vi "main.vi"() -> ()   [LabVIEW 2021]
uses:
  13197e2e-4878-48b7-aae8-aaf27b3d4d67.vi
  0f9acb16-a936-4ed4-a93c-6b467a9371f4.vi
  96cf3d6d-d879-4930-96c0-5a5e60d91763.vi
  Global.vi
  <vilib>/Utility/file.llb/Read Delimited Spreadsheet (DBL).vi
  <vilib>/addons/_NISVFA/_Generation/SoundVib_Generation.lvlib
  <vilib>/measure/NI_MABase.lvlib
panel:
  in  "开始测试":bool
  in  "Stop":bool
  in  "起始频率[Hz]":dbl=1.0 min=1.0 step=100.0
  in  "终止频率[Hz]":dbl=1.0 min=1.0 step=100.0
  in  "信号幅值[V]":dbl min=0.0001 step=0.1
  in  "单次信号时长[s]":dbl
  in  "应用":bool
  in  "Save Button":bool
  in  "Buffer":T1={"# buffers"=4, "Buffer size"=2048, "unit (ms)"=enum."Samples"}
  out "format":cluster{"Rate":i32, "Bits":i32, "Channels":u32}
  out "Waveform Graph":dbl[](graph) caption="Waveform Graph - Dark"
  out "Waveform Graph 3":i32[][](graph)
  out "error out 3":errorcluster
  out "error out":errorcluster
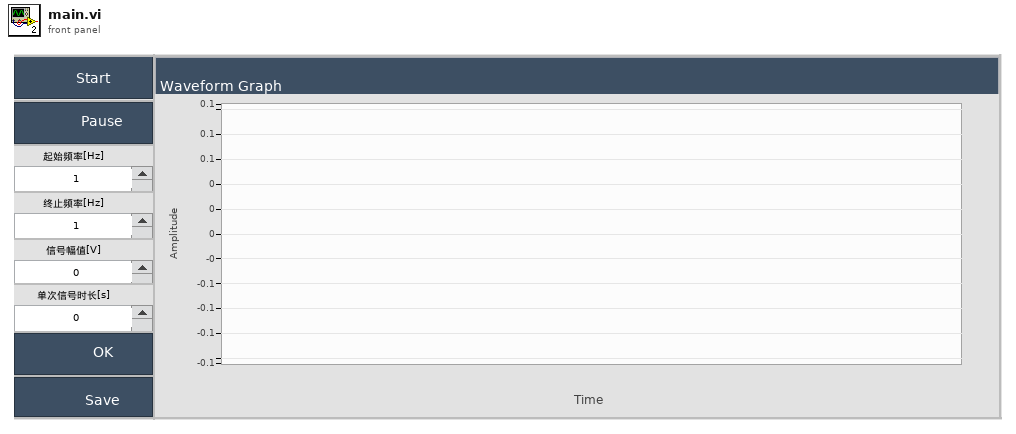
[diagram p1: front panel]
types:
  T1 = cluster{"# buffers":i32, "Buffer size":i32, "unit (ms)":enum16{"time (ms)", "Samples"}}
  T2 = cluster{"slope":dbl, "intercept":dbl, "校准电压值":dbl[]}
  T3 = cluster{"start frequency [Hz]":dbl, "stop frequency [Hz]":dbl}
  T4 = typedef "SoundHandle.ctl" = cluster{"DeviceID":u16, "Samples/buf":u32, "Sampl rate":u32, "Bits/sample":u16, "Channels":u8, "Opened":bool}
  T5 = cluster{"起始频率":dbl, "终止频率":dbl, "信号幅值":dbl, "信号时长":dbl, "重复次数":i32, "扫频模式":bool}
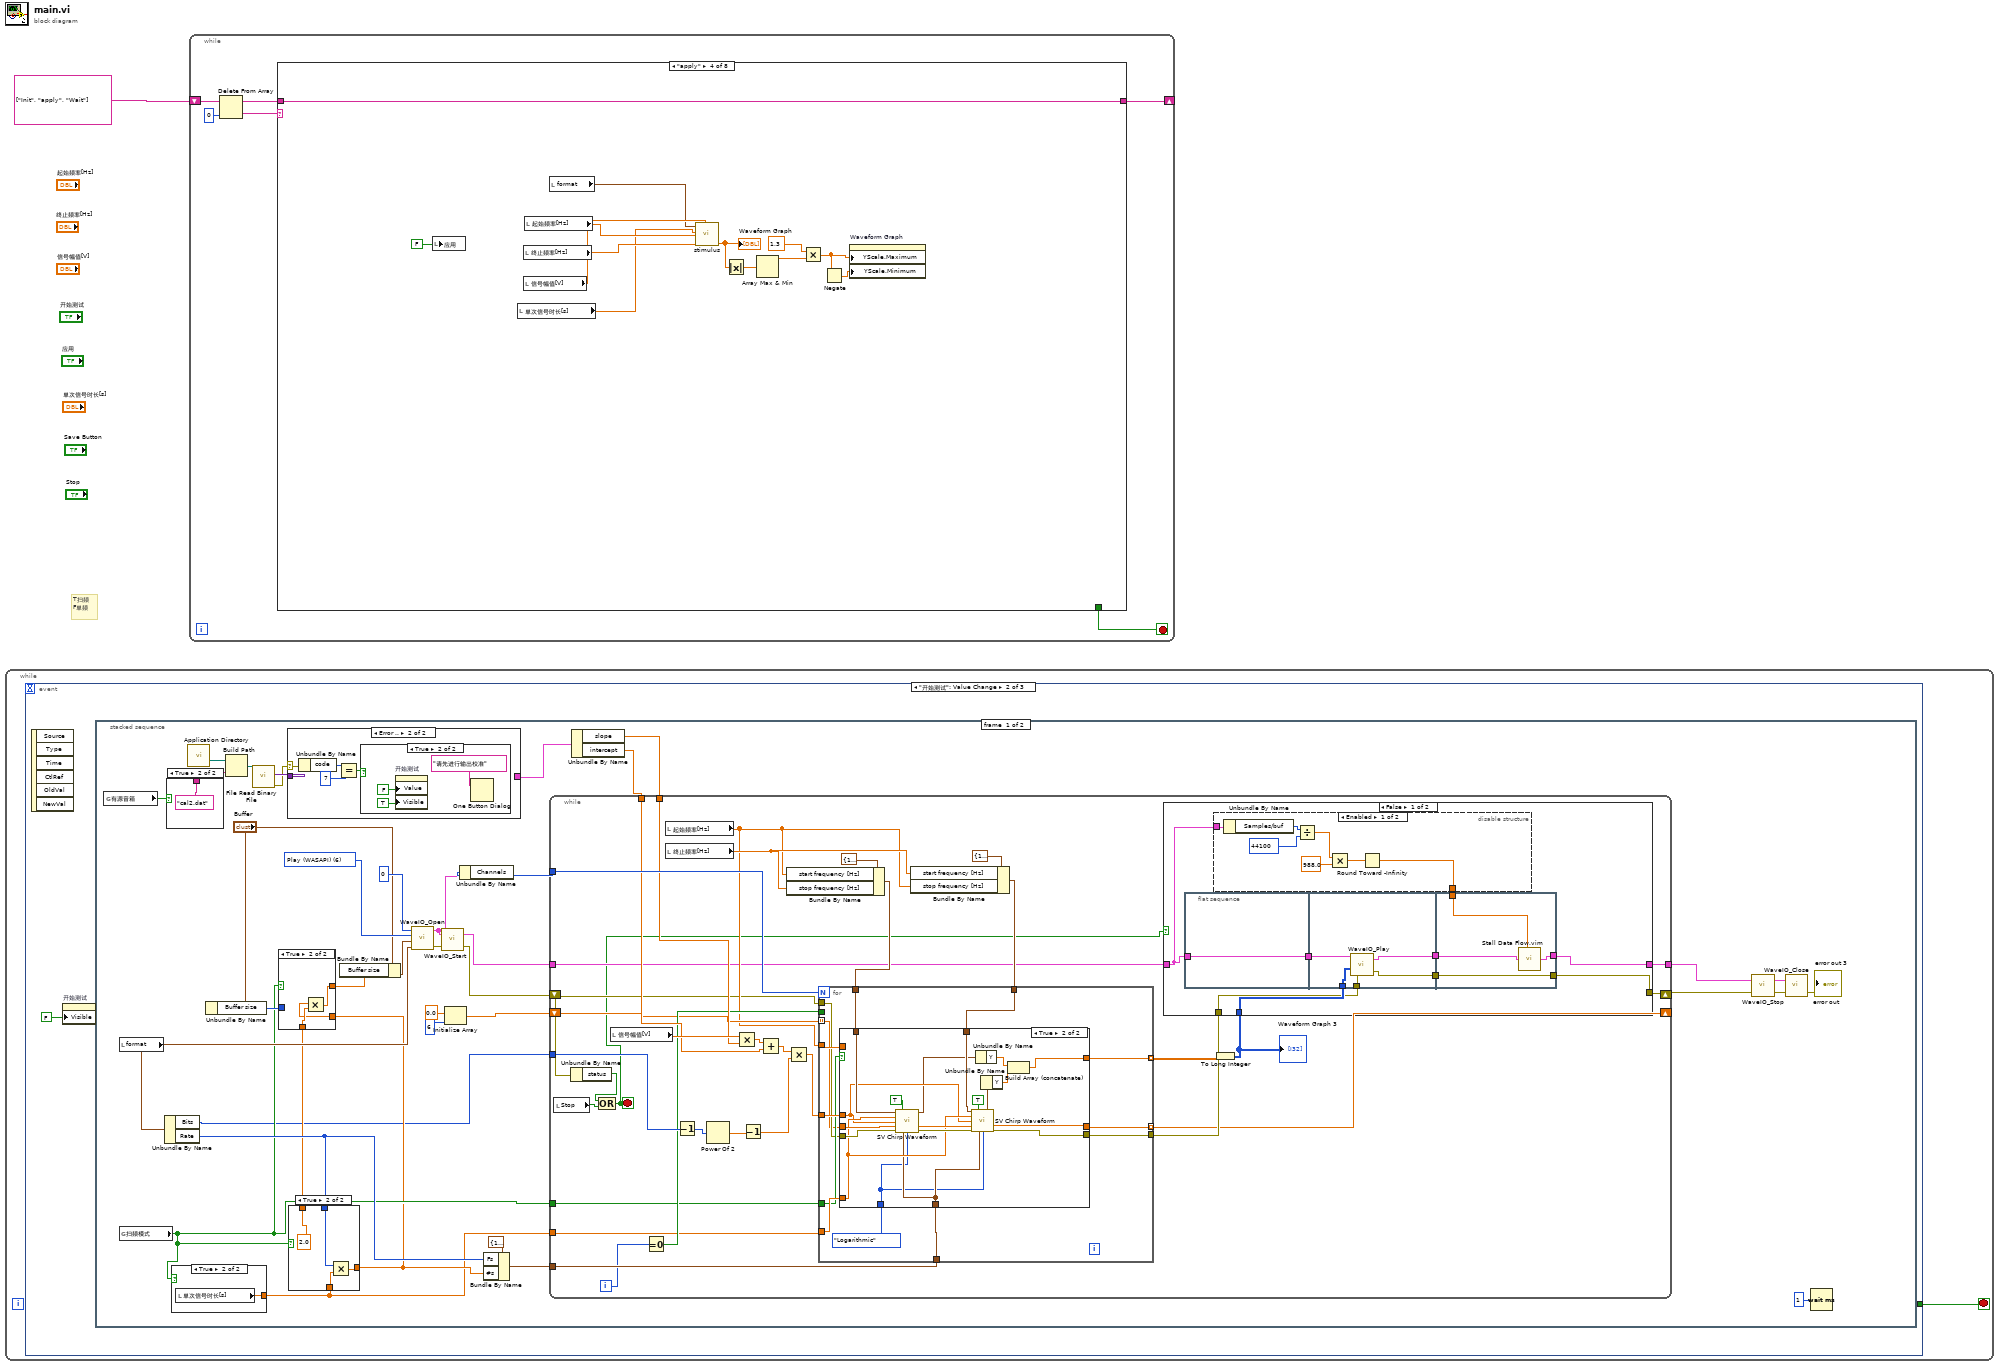
[diagram p0: block diagram]
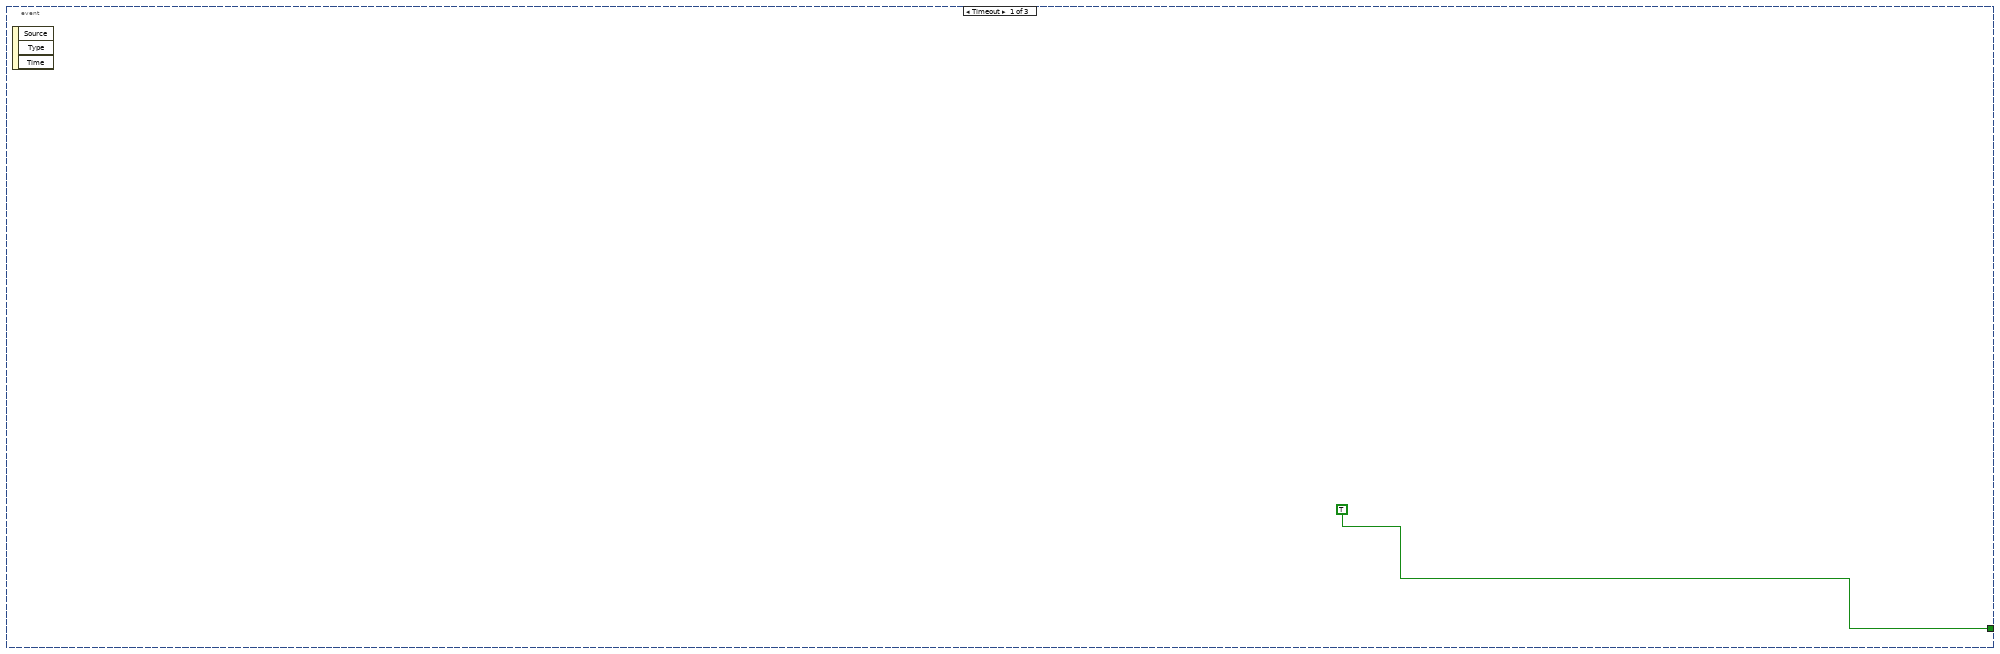
[diagram p2: hidden frame]
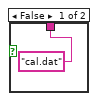
[diagram p3: hidden frame]
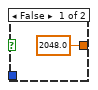
[diagram p4: hidden frame]
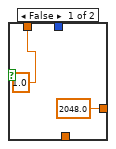
[diagram p5: hidden frame]
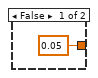
[diagram p6: hidden frame]
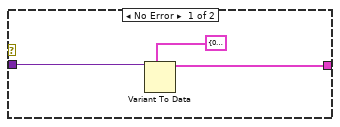
[diagram p7: hidden frame]
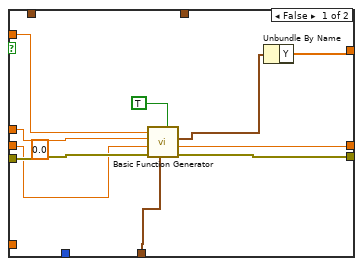
[diagram p11: hidden frame]
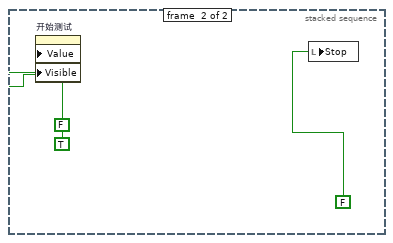
[diagram p12: hidden frame]
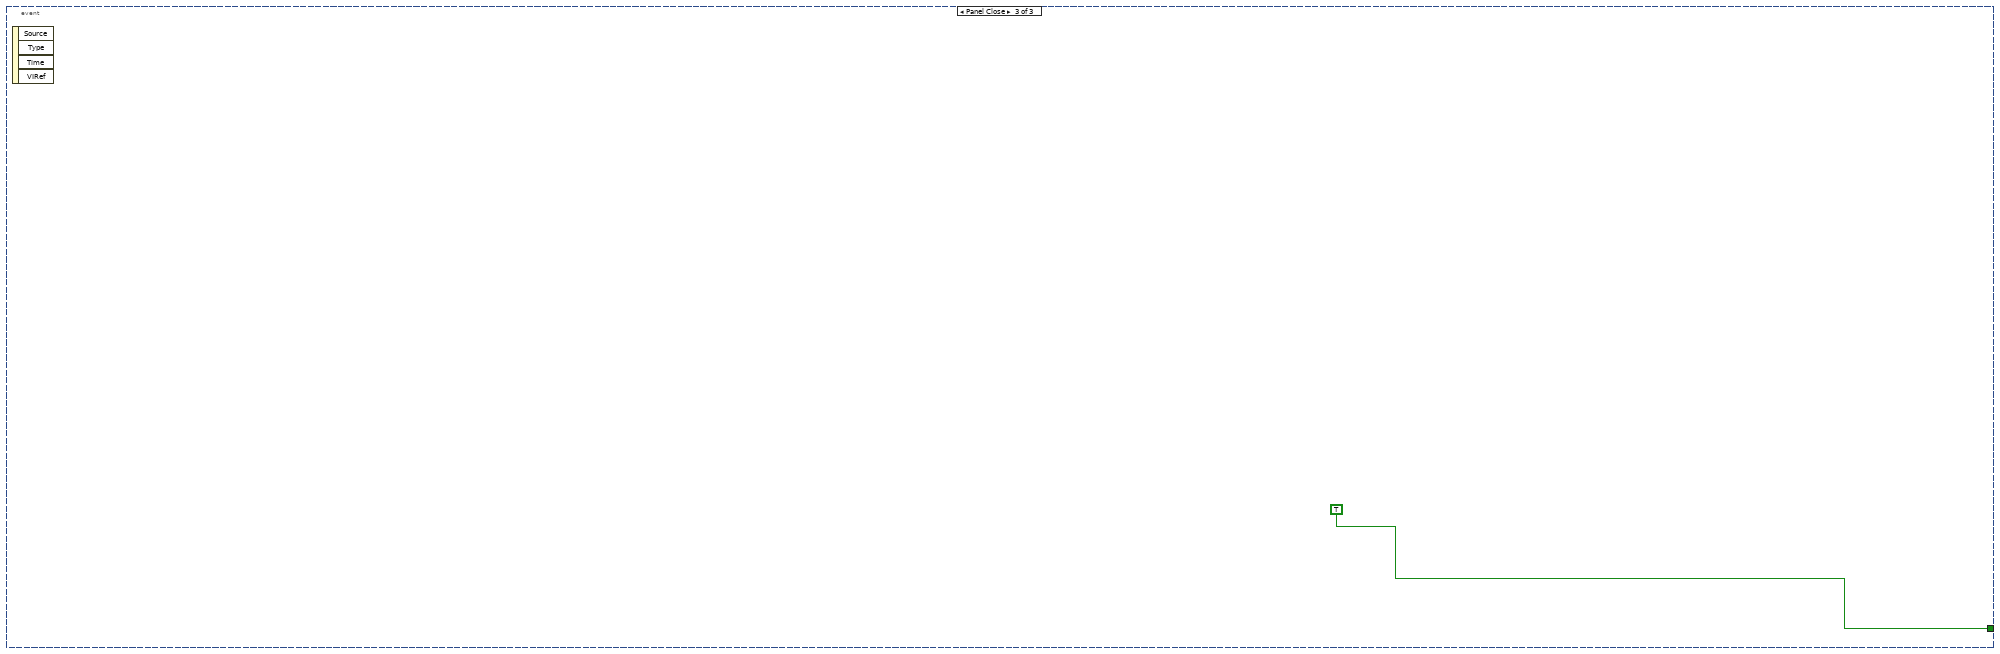
[diagram p13: hidden frame]
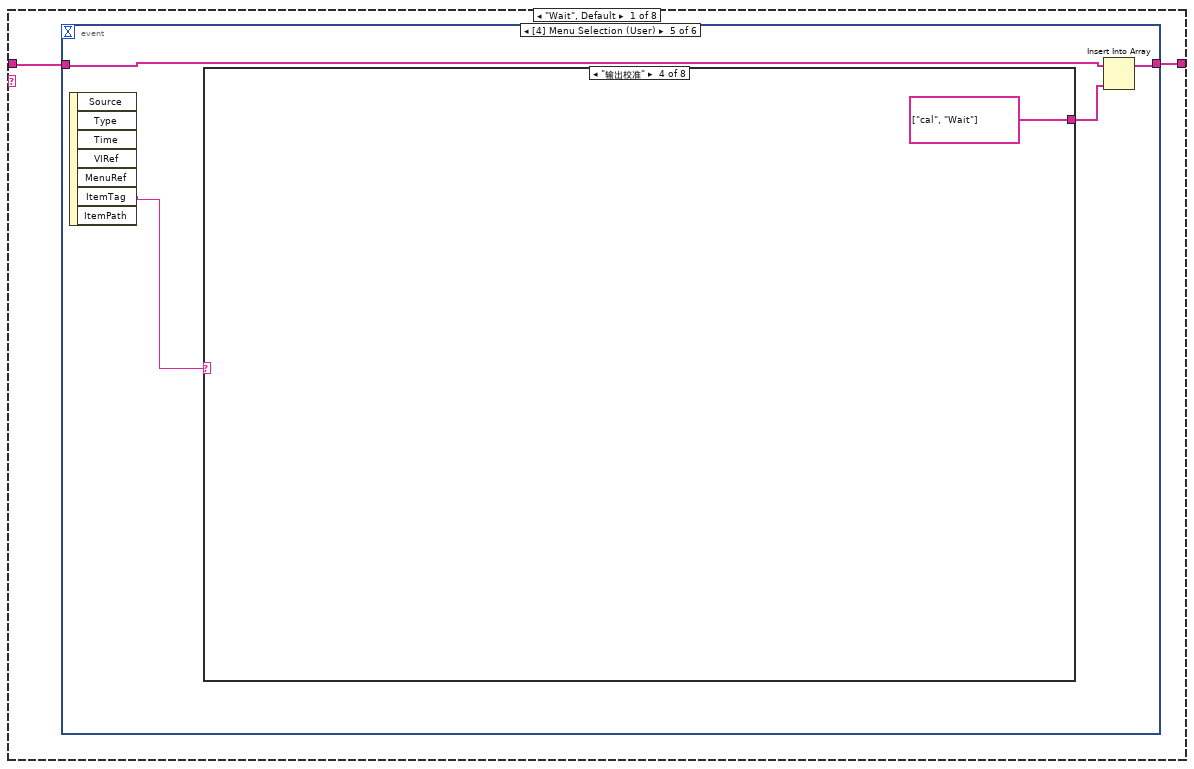
[diagram p14: hidden frame]
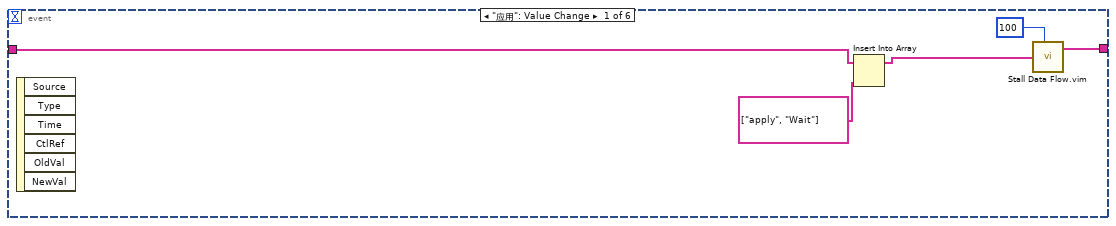
[diagram p15: hidden frame]
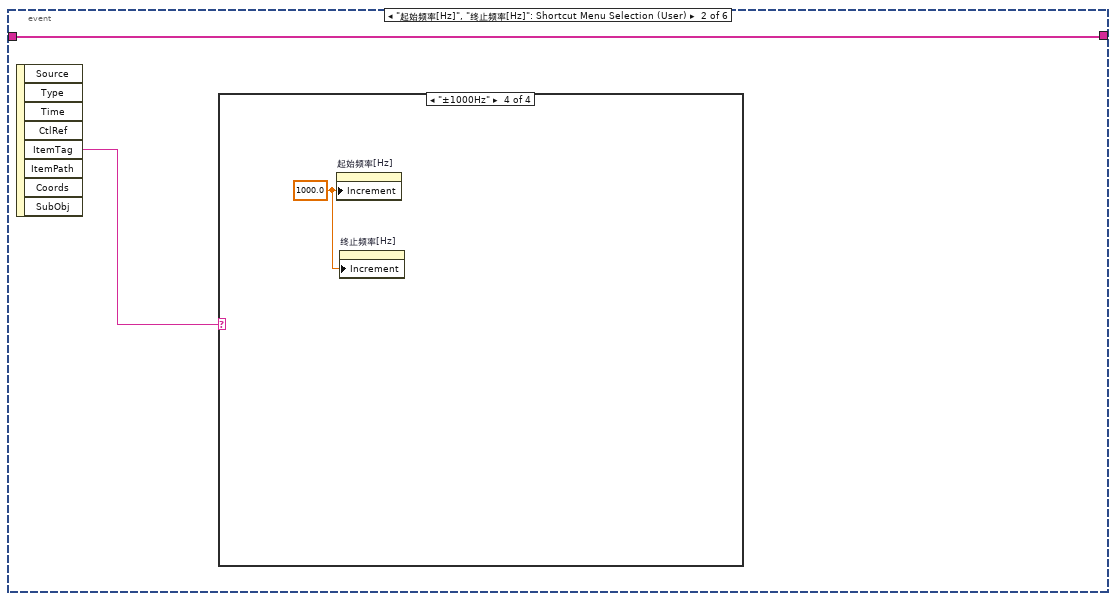
[diagram p16: hidden frame]
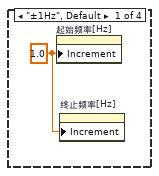
[diagram p17: hidden frame]
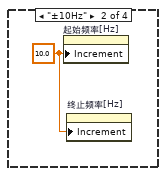
[diagram p18: hidden frame]
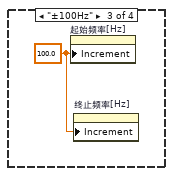
[diagram p19: hidden frame]
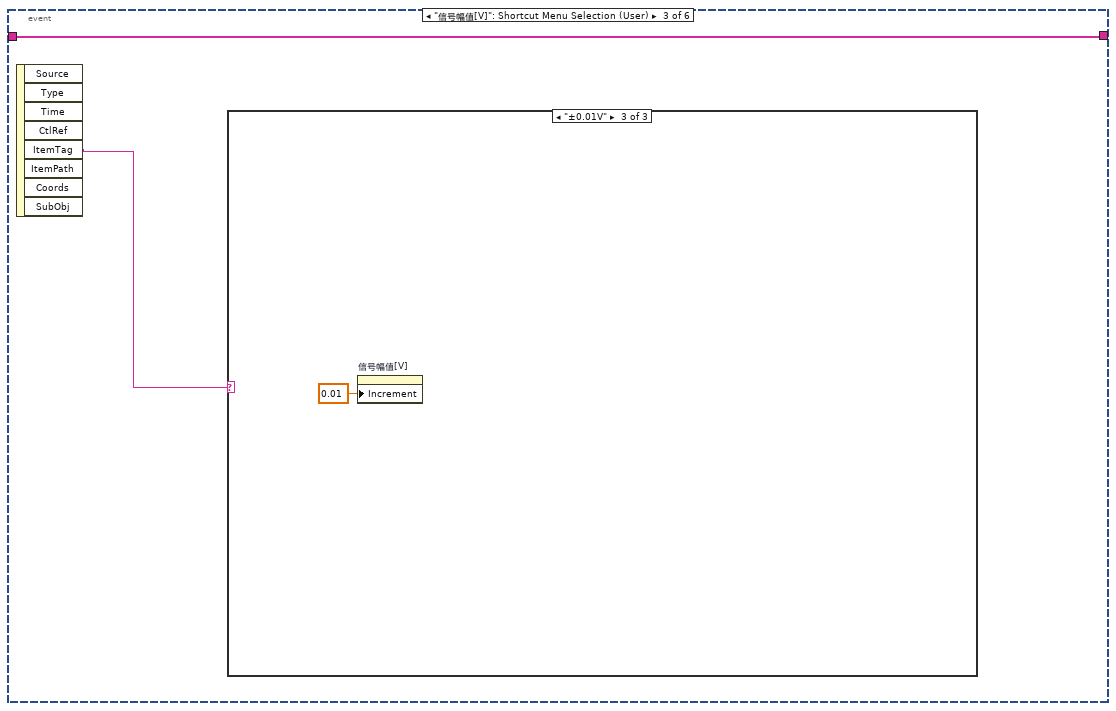
[diagram p20: hidden frame]
diagram:
  # "T扫频\nF单频"
  n1 = while {
    stop <- w2 stop-if-true
    n2 = event shown="[1] \"开始测试\": Value Change" {
      selector: _ -> [_ _ _]
      dyn-events: _ -> [_ _ _]
      timeout: _ -> [_ _ _]
      tunnel: [TRUE ("放弃？") _ TRUE ("放弃？")] -> w2
      event Timeout {
        n3 = event-data() -> ()  [unwired: 1 in, 3 out]
      }
      event "开始测试": Value Change {
        n4 = event-data() -> ()  [unwired: 1 in, 6 out]
        n5 = property on="开始测试" class="Bool (strict)"("Visible"=FALSE) -> ()  [unwired: 2 in, 2 out]
        n6 = stacked-sequence {
          frame #0 {
            w27 = u16 6 items=["Record", "Play", "Loopback", "ASIO input", "ASIO output", "Record (WASAPI)", "Play (WASAPI)", "Record Combi", "Play Combi"] ("device type (Record)")
            n7 = global read "Global.vi" "有源音箱"() -> (w5:bool)
            n8 = local read "format"() -> (w42:cluster{"Rate":i32, "Bits":i32, "Channels":u32})
            n9 = global read "Global.vi" "扫频模式"() -> (w9:bool)
            n10 = Unbundle By Name(w42) -> ("Bits"=w6:i32, "Rate"=w15:i32)
            n11 = case shown="True" w5 {
              tunnel: ["cal.dat" ("名称或相对路径") "cal2.dat" ("名称或相对路径")] -> w26
              frame False {
              }
              frame True {
              }
            }
            n12 = case shown="True" w9 {
              tunnel: [0.05 ("单次信号时长[s]") w57] -> w7
              frame False {
              }
              frame True {
                n13 = local read "单次信号时长[s]"() -> (w57:dbl)
              }
            }
            n14 = call <vilib>:"Application Directory.vi"() -> ("Application Directory"=w25:path)
            n15 = Unbundle By Name("Buffer") -> ("Buffer size"=w10:i32)
            n16 = Build Path(base path=w25, name or relative path=w26) -> (appended path=w24:path)
            n17 = call "File Read Binary File.vi"("file path"=w24) -> ("error Output"=w19:errorcluster, "Variant Output"=w23:variant)  [unwired: 8 in, 1 out]
            n18 = case shown="Error .." w19 {
              selector: w19 -> [_ w64]
              tunnel: w23 -> [w60 _]
              tunnel: [w59 _] -> w22
              frame No Error {
                n19 = Variant To Data(type=T2 {"slope"=0.0, "intercept"=0.0, "校准电压值"=[3.37, 6.73, 10.1, 13.48]}, Variant=w60) -> (data=w59:T2)  [unwired: 1 in, 1 out]
              }
              frame Error {
                n20 = Unbundle By Name(w64) -> ("code"=w63:i32)
                n21 = Equal?(x=w63, y=7) -> (x = y?=w61:bool)
                n22 = case shown="True" w61 {
                  frame False {
                  }
                  frame True {
                    n23 = property on="开始测试" class="Bool (strict)"("Value"=FALSE ("开始测试"), "Visible"=TRUE) -> ()  [unwired: 2 in, 2 out]
                    n24 = One Button Dialog(message="请先进行输出校准") -> ()  [unwired: 1 in, 1 out]
                  }
                }
              }
            }
            n25 = case shown="True" w9 {
              tunnel: [2048.0 w54] -> w8
              tunnel: w7 -> [_ w52]
              tunnel: w15 -> [_ w53]
              tunnel: [1.0 ("x") 2.0 ("x")] -> w11
              frame False {
              }
              frame True {
                n26 = Multiply(x=w53, y=w52) -> (x*y=w54:dbl)
              }
            }
            n27 = case shown="True" w9 {
              tunnel: [2048.0 w47] -> w12
              tunnel: w11 -> [_ w49]
              tunnel: w10 -> [_ _]
              tunnel: w8 -> [_ w48]
              frame False {
              }
              frame True {
                n28 = Multiply(x=w48, y=w49) -> (x*y=w47:dbl)
              }
            }
            n29 = Bundle By Name(cluster="Buffer", "Buffer size"=w12) -> (w14:T1)
            n30 = call "WaveIO_Open.vi"("idev"=u32 0, "device type (Record)"=w27, "Buffer Config"=w14, "Format (44kHz, 16Bit, stereo)"=w42) -> ("Sound Handle Out"=w38:T4, "error out"=w35:errorcluster)  [unwired: 3 in]
            n31 = call "WaveIO_Start.vi"("error in (no error)"=w35, "Handle"=w38) -> ("error out"=w34:errorcluster, "Handle Out"=w33:T4)
            n32 = Initialize Array(0.0 ("element"), 6 ("dimension size")) -> (w16:dbl[])
            n33 = Unbundle By Name(w38) -> ("Channels"=w39:u8)
            n34 = Bundle By Name(cluster=cluster{"Fs":dbl, "#s":dbl} {"Fs"=1000.0, "#s"=1000.0} ("sampling info"), "Fs"=w15, "#s"=w8) -> (w32:cluster{"Fs":dbl, "#s":dbl})
            n35 = Unbundle By Name(w22) -> ("slope"=w21:dbl, "intercept"=w20:dbl)
            n36 = while {
              shift-right: [w95] -> w36
              shift-left: w34 -> [w70]
              tunnel: w33 -> [w73]
              tunnel: [w100] -> w29
              tunnel: w32 -> [w101]
              tunnel: w6 -> [w99]
              tunnel: w39 -> [w94]
              tunnel: w21 -> [w88]
              tunnel: w20 -> [w86]
              tunnel: w9 -> [w82]
              shift-right: [w79] -> _
              shift-left: w16 -> [w80]
              tunnel: w7 -> [w78]
              i -> [w84]
              stop <- w68 stop-if-true
              n37 = local read "Stop"() -> (w92:bool)
              n38 = Unbundle By Name(w70) -> ("status"=w93:bool)
              n39 = Compound Arithmetic op=OR(w93, w92) -> (w68:bool)
              n40 = local read "信号幅值[V]"() -> (w89:dbl)
              n41 = Equal To 0?(x=w84) -> (x = 0?=w83:bool)
              n42 = local read "起始频率[Hz]"() -> (w75:dbl)
              n43 = local read "终止频率[Hz]"() -> (w76:dbl)
              n44 = Decrement(x=w99) -> (x-1=w98:i32)
              n45 = Power Of 2(x=w98) -> (2^x=w72:dbl)
              n46 = Multiply(x=w89, y=w88) -> (x*y=w87:dbl)
              n47 = Decrement(x=w72) -> (x-1=w71:dbl)
              n48 = Add(x=w87, y=w86) -> (x+y=w85:dbl)
              n49 = Bundle By Name(cluster=T3 {"start frequency [Hz]"=10.0, "stop frequency [Hz]"=10000.0} ("frequency range"), "start frequency [Hz]"=w75, "stop frequency [Hz]"=w76) -> (w90:T3)
              n50 = Multiply(x=w85, y=w71) -> (x*y=w97:dbl)
              n51 = Bundle By Name(cluster=T3 {"start frequency [Hz]"=10.0, "stop frequency [Hz]"=10000.0} ("frequency range"), "start frequency [Hz]"=w76, "stop frequency [Hz]"=w75) -> (w74:T3)
              n52 = for {
                N: w94 -> [_]
                tunnel: w101 -> [w142]
                tunnel: w97 -> [w141]
                tunnel: [w130] -> w69 mode=indexing
                tunnel: w90 -> [w140]
                tunnel: w78 -> [w139]
                tunnel: w83 -> [_]
                tunnel: w82 -> [w137]
                tunnel: w75 -> [w136]
                tunnel: w70 -> [w135]
                tunnel: [w134] -> w81
                tunnel: w80 -> [w133] mode=indexing
                tunnel: [w132] -> w79 mode=indexing
                tunnel: w74 -> [w131]
                n53 = case shown="True" w137 {
                  tunnel: w142 -> [w148 w155]
                  tunnel: w141 -> [w151 w163]
                  tunnel: w140 -> [_ w170]
                  tunnel: w139 -> [_ w164]
                  tunnel: enum16{"Linear", "Logarithmic"}."Logarithmic" ("frequency spacing") -> [_ w154]
                  tunnel: w136 -> [w152 _]
                  tunnel: w135 -> [w150 w169]
                  tunnel: [w149 w168] -> w134
                  tunnel: w133 -> [w146 w166]
                  tunnel: [w147 w160] -> w132
                  tunnel: w131 -> [_ w162]
                  tunnel: [w143 w153] -> w130
                  frame False {
                    (unwired) 0.0 ("phase")
                    n54 = call <vilib>:"Basic Function Generator.vi"("reset signal"=TRUE, "sampling info"=w148, "error in (no error)"=w150, "phase"=w146, "amplitude"=w151, "frequency"=w152) -> ("error out"=w149:errorcluster, "phase out"=w147:dbl, "signal out"=w145:waveform(dbl))  [unwired: 3 in]
                    n55 = Unbundle By Name(w145) -> ("Y"=w143:dbl[])
                  }
                  frame True {
                    n56 = call <vilib>:"SV Chirp Waveform.vi"("frequency range"=w170, "reset signal (F)"=TRUE, "chirp duration [s]"=w164, "amplitude"=w163, "phase in [deg]"=w166, "error in (no error)"=w169, "sampling info"=w155, "frequency spacing"=w154) -> ("chirp signal"=w159:waveform(dbl), "phase out [deg]"=w165:dbl, "error out"=w168:errorcluster)  [unwired: 5 in]
                    n57 = call <vilib>:"SV Chirp Waveform.vi"("frequency range"=w162, "reset signal (F)"=TRUE, "chirp duration [s]"=w164, "amplitude"=w163, "phase in [deg]"=w165, "sampling info"=w155, "frequency spacing"=w154) -> ("chirp signal"=w158:waveform(dbl), "phase out [deg]"=w160:dbl)  [unwired: 6 in, 1 out]
                    n58 = Unbundle By Name(w159) -> ("Y"=w157:dbl[])
                    n59 = Unbundle By Name(w158) -> ("Y"=w156:dbl[])
                    n60 = Build Array (concatenate)(w157, w156) -> (w153:dbl[])
                  }
                }
              }
              n61 = To Long Integer(number=w69) -> (32bit integer=w96:i32[][])
              "Waveform Graph 3" <- w96
              n62 = case shown="False" w68 {
                tunnel: [w103 w129] -> w100
                tunnel: w96 -> [w110 _]
                tunnel: [w109 w128] -> w95
                tunnel: w81 -> [w108 w128]
                tunnel: w73 -> [w105 w129]
                frame False {
                  n63 = flat-sequence {
                    tunnel: w105 -> [w111]
                    tunnel: [w111] -> w104
                    tunnel: w110 -> [w116]
                    tunnel: w108 -> [w114]
                    tunnel: [w115] -> w107
                    tunnel: [w113] -> w106
                    tunnel: w104 -> [w112]
                    tunnel: w107 -> [w120]
                    tunnel: w106 -> [w118]
                    tunnel: w102 -> [w117]
                    tunnel: [w120] -> w109
                    tunnel: [w119] -> w103
                    frame #0 {
                    }
                    frame #1 {
                      n64 = call "WaveIO_Play.vi"("error in (no error)"=w114, "data"=w116, "Handle"=w112) -> ("error out"=w115:errorcluster, "Handle Out"=w113:T4)  [unwired: 1 in]
                    }
                    frame #2 {
                      n65 = call "Stall Data Flow.vim"("value in"=w118, "milliseconds to wait"=w117) -> ("value out"=w119:T4)  [unwired: 1 out]
                    }
                  }
                  n66 = disable-structure shown="Enabled" {
                    disable-tunnel: w105 -> [w125 _]
                    disable-tunnel: [w121 _] -> w102
                    frame Enabled {
                      n67 = Unbundle By Name(w125) -> ("Samples/buf"=w127:u32)
                      n68 = Divide(x=w127, y=u32 44100) -> (x/y=w124:dbl)
                      n69 = Multiply(x=w124, y=988.0) -> (x*y=w122:dbl)
                      n70 = Round Toward -Infinity(1:w122) -> (0:w121:dbl)
                    }
                    frame Disabled {
                    }
                  }
                }
                frame True {
                }
              }
            }
            n71 = call "WaveIO_Stop.vi"("error in (no error)"=w36, "Handle"=w29) -> ("error out"=w30:errorcluster, "Handle Out"=w28:T4)
            n72 = call "WaveIO_Close.vi"("error in (no error)"=w30, "Handle"=w28) -> ("error out"=→"error out 3":errorcluster)  [unwired: 1 out]
            n73 = Wait (ms)(milliseconds to wait=u32 1) -> ()  [unwired: 1 out]
            n74 = Wait (ms)(milliseconds to wait=u32 1) -> ()  [unwired: 1 out]
          }
          frame #1 {
            n75 = property on="开始测试" class="Bool (strict)"("Value"=FALSE ("开始测试"), "Visible"=TRUE) -> ()  [unwired: 2 in, 2 out]
            n76 = local write "Stop"(FALSE ("Stop")) -> ()
          }
        }
      }
      event Panel Close {
        n77 = event-data() -> ()  [unwired: 1 in, 4 out]
      }
    }
  }
  n78 = while {
    shift-right: [w176] -> _
    shift-left: string[] ["Init", "apply", "Wait"] -> [w180]
    stop <- w175 stop-if-true
    n79 = Delete From Array(array=w180, index=0 ("索引")) -> (deleted portion=w178:string, array with subset deleted=w177:string[])  [unwired: 1 in]
    n80 = case shown="\"apply\"" w178 {
      tunnel: w177 -> [w181 w224 w232 w251 w257 w294 w359 w388]
      tunnel: [w182 w224 w232 w251 w257 w295 w359 w388] -> w176
      tunnel: [_ _ _ _ _ _ TRUE _] -> w175
      frame "Wait", Default {
        n81 = event shown="[4] Menu Selection (User)" {
          selector: _ -> [_ _ _ _ _ _]
          dyn-events: _ -> [_ _ _ _ _ _]
          timeout: _ -> [_ _ _ _ _ _]
          tunnel: [w187 w189 w194 w203 w204 w221] -> w182
          tunnel: w181 -> [w185 w189 w194 w201 w206 w223]
          event "应用": Value Change {
            n82 = event-data() -> ()  [unwired: 1 in, 6 out]
            n83 = Insert Into Array(array=w185, new element=string[] ["apply", "Wait"]) -> (w183:string[])  [unwired: 1 in]
            n84 = call "Stall Data Flow.vim"("value in"=w183, "milliseconds to wait"=u32 100) -> ("value out"=w187:string[])  [unwired: 1 out]
          }
          event "起始频率[Hz]", "终止频率[Hz]": Shortcut Menu Selection (User) {
            n85 = event-data() -> ("ItemTag"=w188:string)  [unwired: 1 in, 7 out]
            n86 = case shown="\"±1000Hz\"" w188 {
              frame "±1Hz", Default {
                w190 = 1.0 ("Data Entry Limits:Increment")
                n87 = property on="起始频率[Hz]" class="DigNum (strict)"("Increment"=w190) -> ()  [unwired: 2 in, 2 out]
                n88 = property on="终止频率[Hz]" class="DigNum (strict)"("Increment"=w190) -> ()  [unwired: 2 in, 2 out]
              }
              frame "±10Hz" {
                w191 = 10.0 ("Data Entry Limits:Increment")
                n89 = property on="起始频率[Hz]" class="DigNum (strict)"("Increment"=w191) -> ()  [unwired: 2 in, 2 out]
                n90 = property on="终止频率[Hz]" class="DigNum (strict)"("Increment"=w191) -> ()  [unwired: 2 in, 2 out]
              }
              frame "±100Hz" {
                w192 = 100.0 ("Data Entry Limits:Increment")
                n91 = property on="起始频率[Hz]" class="DigNum (strict)"("Increment"=w192) -> ()  [unwired: 2 in, 2 out]
                n92 = property on="终止频率[Hz]" class="DigNum (strict)"("Increment"=w192) -> ()  [unwired: 2 in, 2 out]
              }
              frame "±1000Hz" {
                w193 = 1000.0 ("Data Entry Limits:Increment")
                n93 = property on="起始频率[Hz]" class="DigNum (strict)"("Increment"=w193) -> ()  [unwired: 2 in, 2 out]
                n94 = property on="终止频率[Hz]" class="DigNum (strict)"("Increment"=w193) -> ()  [unwired: 2 in, 2 out]
              }
            }
          }
          event "信号幅值[V]": Shortcut Menu Selection (User) {
            n95 = event-data() -> ("ItemTag"=w195:string)  [unwired: 1 in, 7 out]
            n96 = case shown="\"±0.01V\"" w195 {
              frame "±1V", Default {
                n97 = property on="信号幅值[V]" class="DigNum (strict)"("Increment"=1.0 ("Data Entry Limits:Increment")) -> ()  [unwired: 2 in, 2 out]
              }
              frame "±0.1V" {
                n98 = property on="信号幅值[V]" class="DigNum (strict)"("Increment"=0.1 ("Data Entry Limits:Increment")) -> ()  [unwired: 2 in, 2 out]
              }
              frame "±0.01V" {
                n99 = property on="信号幅值[V]" class="DigNum (strict)"("Increment"=0.01 ("Data Entry Limits:Increment")) -> ()  [unwired: 2 in, 2 out]
              }
            }
          }
          event "Save Button": Value Change {
            n100 = event-data() -> ()  [unwired: 1 in, 6 out]
            n101 = Insert Into Array(array=w201, new element=string[] ["save", "Wait"]) -> (w199:string[])  [unwired: 1 in]
            n102 = call "Stall Data Flow.vim"("value in"=w199, "milliseconds to wait"=u32 100) -> ("value out"=w203:string[])  [unwired: 1 out]
          }
          event Menu Selection (User) {
            n103 = event-data() -> ("ItemTag"=w207:string)  [unwired: 1 in, 6 out]
            n104 = case shown="\"输出校准\"" w207 {
              tunnel: [_ string[] ["signal out", "Wait"] string[] ["signal in", "Wait"] string[] ["cal", "Wait"] _ _ _ _] -> w205
              frame Default {
              }
              frame "扫频信号导出" {
              }
              frame "扫频信号导入" {
              }
              frame "输出校准" {
              }
              frame "单频" {
                n105 = property on="单次信号时长[s]" class="DigNum (strict)"("Visible"=FALSE) -> ()  [unwired: 2 in, 2 out]
                n106 = property on="终止频率[Hz]" class="DigNum (strict)"("Visible"=FALSE) -> ()  [unwired: 2 in, 2 out]
                n107 = global write "Global.vi" "扫频模式"(FALSE ("扫频模式")) -> ()
                n108 = property on="起始频率[Hz]" class="DigNum (strict)"("Caption.Text"="单频频率[Hz]") -> ()  [unwired: 2 in, 2 out]
              }
              frame "有源音箱" {
                n109 = global write "Global.vi" "有源音箱"(TRUE ("有源音箱")) -> ()
              }
              frame "其它" {
                n110 = global write "Global.vi" "有源音箱"(FALSE ("有源音箱")) -> ()
              }
              frame "扫频" {
                n111 = property on="单次信号时长[s]" class="DigNum (strict)"("Visible"=TRUE) -> ()  [unwired: 2 in, 2 out]
                n112 = property on="终止频率[Hz]" class="DigNum (strict)"("Visible"=TRUE) -> ()  [unwired: 2 in, 2 out]
                n113 = global write "Global.vi" "扫频模式"(TRUE ("扫频模式")) -> ()
                n114 = property on="起始频率[Hz]" class="DigNum (strict)"("Caption.Text"="起始频率[Hz]") -> ()  [unwired: 2 in, 2 out]
              }
            }
            n115 = Insert Into Array(array=w206, new element=w205) -> (w204:string[])  [unwired: 1 in]
          }
          event Panel Close? {
            n116 = event-data() -> ()  [unwired: 1 in, 4 out]
            n117 = Insert Into Array(array=w223, new element="Exit" ("new element/subarray")) -> (w221:string[])  [unwired: 1 in]
            n118 = event-data() -> ()  [unwired: 2 in, 1 out]
          }
        }
      }
      frame "cal" {
        n119 = local read "单次信号时长[s]"() -> (w230:dbl)
        n120 = local read "起始频率[Hz]"() -> (w228:dbl)
        n121 = local read "终止频率[Hz]"() -> (w229:dbl)
        n122 = local read "信号幅值[V]"() -> (w227:dbl)
        n123 = local read "Buffer"() -> (w226:T1)
        n124 = local read "format"() -> (w225:cluster{"Rate":i32, "Bits":i32, "Channels":u32})
        n125 = call "calibration.vi"("信号时长[s]"=w230, "Buffer"=w226, "终止频率[Hz]"=w229, "起始频率[Hz]"=w228, "信号幅值[V]"=w227, "format"=w225) -> ()  [unwired: 10 in]
      }
      frame "save" {
        n126 = local read "单次信号时长[s]"() -> (w238:dbl)
        n127 = global read "Global.vi" "扫频模式"() -> (w231:bool)
        n128 = local read "终止频率[Hz]"() -> (w240:dbl)
        n129 = local read "信号幅值[V]"() -> (w239:dbl)
        n130 = local read "起始频率[Hz]"() -> (w241:dbl)
        n131 = local write "Save Button"(FALSE ("应用")) -> ()
        n132 = Bundle By Name(cluster=T5 {"起始频率"=0.0, "终止频率"=0.0, "信号幅值"=0.0, "信号时长"=0.0, "重复次数"=3, "扫频模式"=TRUE}, "起始频率"=w241, "终止频率"=w240, "信号幅值"=w239, "信号时长"=w238, "扫频模式"=w231) -> (w237:T5)
        n133 = call <vilib>:"Application Directory.vi"() -> ("Application Directory"=w243:path)
        n134 = Build Path(base path=w243, name or relative path="main.dat" ("名称或相对路径")) -> (appended path=w242:path)
        n135 = call "File Write to Variant.vi"("替换提示"=FALSE, "Input Data"=w237, "Path to Write"=w242) -> ()  [unwired: 4 in, 5 out]
      }
      frame "apply" {
        n136 = local write "应用"(FALSE ("应用")) -> ()
        n137 = local read "单次信号时长[s]"() -> (w252:dbl)
        n138 = local read "终止频率[Hz]"() -> (w255:dbl)
        n139 = local read "信号幅值[V]"() -> (w254:dbl)
        n140 = local read "起始频率[Hz]"() -> (w256:dbl)
        n141 = local read "format"() -> (w253:cluster{"Rate":i32, "Bits":i32, "Channels":u32})
        n142 = call "stimulus.vi"("幅值(V)"=w254, "stop frequency [Hz]"=w255, "start frequency [Hz]"=w256, "信号时长"=w252, "Format"=w253) -> ("sti"=w250:dbl[])  [unwired: 4 in, 2 out]
        "Waveform Graph" <- w250
        n143 = Absolute Value(x=w250) -> (abs(x)=w249:dbl[])
        n144 = Array Max & Min(array=w249) -> (max value=w248:dbl)  [unwired: 3 out]
        n145 = Multiply(x=1.3, y=w248) -> (x*y=w245:dbl)
        n146 = Negate(x=w245) -> (-x=w246:dbl)
        n147 = property on="Waveform Graph" class="WFGraph (strict)"("YScale.Maximum"=w245, "YScale.Minimum"=w246) -> ()  [unwired: 2 in, 2 out]
      }
      frame "signal out" {
        n148 = stacked-sequence {
          frame #0 {
            n149 = global read "Global.vi" "扫频模式"() -> (w258:bool)
            n150 = case shown="True" w258 {
              frame True {
                w259 = "Hz" ("string")
                w262 = i16 2 ("precision (6)")
                w261 = "-" ("string")
                w263 = i16 0 ("precision (6)")
                n151 = local read "信号幅值[V]"() -> (w270:dbl)
                n152 = local read "单次信号时长[s]"() -> (w267:dbl)
                n153 = local read "起始频率[Hz]"() -> (w274:dbl)
                n154 = local read "终止频率[Hz]"() -> (w273:dbl)
                n155 = local read "format"() -> (w277:cluster{"Rate":i32, "Bits":i32, "Channels":u32})
                n156 = call "stimulus.vi"("幅值(V)"=w270, "stop frequency [Hz]"=w273, "start frequency [Hz]"=w274, "信号时长"=w267, "Format"=w277) -> ("sti"=w276:dbl[])  [unwired: 4 in, 2 out]
                n157 = Number To Fractional String(number=w274, precision (6)=w263) -> (F-format string=w272:string)  [unwired: 2 in]
                n158 = Number To Fractional String(number=w273, precision (6)=w263) -> (F-format string=w271:string)  [unwired: 2 in]
                n159 = Number To Fractional String(number=w270, precision (6)=w262) -> (F-format string=w269:string)  [unwired: 2 in]
                n160 = Number To Fractional String(number=w267, precision (6)=w262) -> (F-format string=w266:string)  [unwired: 2 in]
                n161 = Concatenate Strings(w272, w259, w261, w271, w259, w261, w269, "V" ("string"), w261, w266, "s" ("string"), ".txt" ("string")) -> (w264:string)
                n162 = call "save_wav_as_txt.vi"("文件夹名"="signal", "txt名"=w264, "wav"=w276) -> ()  [unwired: 9 in]
              }
              frame False {
                n163 = local read "信号幅值[V]"() -> (w286:dbl)
                n164 = local read "起始频率[Hz]"() -> (w288:dbl)
                n165 = local read "format"() -> (w291:cluster{"Rate":i32, "Bits":i32, "Channels":u32})
                n166 = call "stimulus.vi"("幅值(V)"=w286, "start frequency [Hz]"=w288, "Format"=w291) -> ("sti"=w290:dbl[])  [unwired: 6 in, 2 out]
                n167 = Number To Fractional String(number=w288, precision (6)=i16 0) -> (F-format string=w287:string)  [unwired: 2 in]
                n168 = Number To Fractional String(number=w286, precision (6)=i16 2) -> (F-format string=w285:string)  [unwired: 2 in]
                n169 = Concatenate Strings(w287, "Hz" ("string"), "-" ("string"), w285, "V" ("string"), ".txt" ("string")) -> (w283:string)
                n170 = call "save_wav_as_txt.vi"("文件夹名"="signal", "txt名"=w283, "wav"=w290) -> ()  [unwired: 9 in]
              }
            }
          }
          frame #1 {
            n171 = One Button Dialog(message="信号已导出") -> ()  [unwired: 1 in, 1 out]
          }
        }
      }
      frame "signal in" {
        n172 = global read "Global.vi" "扫频模式"() -> (w296:bool)
        n173 = case shown="False" w296 {
          frame True {
            w311 = "-" ("regular expression")
            n174 = call <vilib>:"Application Directory.vi"() -> ("Application Directory"=w327:path)
            n175 = Build Path(base path=w327, name or relative path="signal") -> (appended path=w325:path)
            n176 = call "File Dialog"("start path"=w325, "prompt"="选择信号") -> ("selected path"=w323:path, "error out"=w299:errorcluster)  [unwired: 10 in, 2 out]
            n177 = case shown="No Error" w299 {
              tunnel: w323 -> [w330 _]
              tunnel: [w329 _] -> w322
              tunnel: [w328 _] -> w298
              frame No Error {
                n178 = call-poly <vilib>:"Read Delimited Spreadsheet.vi"("file path (dialog if empty)"=w330, "format (%.3f)"="%.9f", "transpose? (F)"=TRUE) -> ("new file path (Not A Path if cancelled)"=w329:path, "first row"=w328:dbl[])  [unwired: 7 in, 4 out]
              }
              frame Error {
              }
            }
            n179 = Strip Path(path=w322) -> (name=w321:string)  [unwired: 1 out]
            n180 = Absolute Value(x=w298) -> (abs(x)=w304:dbl[])
            n181 = Match Pattern(string=w321, regular expression=w311) -> (before substring=w320:string, after substring=w318:string)  [unwired: 1 in, 2 out]
            n182 = property on="Waveform Graph" class="WFGraph (strict)"("Value"=w298) -> (error out=w297:errorcluster)  [unwired: 2 in, 1 out]
            n183 = Array Max & Min(array=w304) -> (max value=w303:dbl)  [unwired: 3 out]
            n184 = Match Pattern(string=w318, regular expression=w311) -> (before substring=w317:string, after substring=w315:string)  [unwired: 1 in, 2 out]
            n185 = Fract/Exp String To Number(string=w320) -> (number=w319:dbl)  [unwired: 3 in, 1 out]
            n186 = Multiply(x=1.3, y=w303) -> (x*y=w300:dbl)
            n187 = Match Pattern(string=w315, regular expression=w311) -> (before substring=w310:string, after substring=w312:string)  [unwired: 1 in, 2 out]
            n188 = Negate(x=w300) -> (-x=w301:dbl)
            n189 = Fract/Exp String To Number(string=w317) -> (number=w316:dbl)  [unwired: 3 in, 1 out]
            n190 = Match Pattern(string=w312, regular expression=w311) -> (before substring=w307:string)  [unwired: 1 in, 3 out]
            n191 = property on="Waveform Graph" class="WFGraph (strict)"(error in=w297, "YScale.Maximum"=w300, "YScale.Minimum"=w301) -> ()  [unwired: 1 in, 2 out]
            n192 = Match Pattern(string=w310, regular expression="V") -> (before substring=w308:string)  [unwired: 1 in, 3 out]
            n193 = local write "终止频率[Hz]"(w316) -> ()
            n194 = local write "起始频率[Hz]"(w319) -> ()
            n195 = Match Pattern(string=w307, regular expression="s") -> (before substring=w305:string)  [unwired: 1 in, 3 out]
            n196 = Fract/Exp String To Number(string=w308) -> (number=w314:dbl)  [unwired: 3 in, 1 out]
            n197 = local write "信号幅值[V]"(w314) -> ()
            n198 = Fract/Exp String To Number(string=w305) -> (number=w313:dbl)  [unwired: 3 in, 1 out]
            n199 = local write "单次信号时长[s]"(w313) -> ()
          }
          frame False {
            w342 = "-" ("regular expression")
            n200 = call <vilib>:"Application Directory.vi"() -> ("Application Directory"=w353:path)
            n201 = Build Path(base path=w353, name or relative path="signal") -> (appended path=w351:path)
            n202 = call "File Dialog2"("start path"=w351, "prompt"="选择信号") -> ("selected path"=w349:path, "error out"=w336:errorcluster)  [unwired: 10 in, 2 out]
            n203 = case shown="Error .." w336 {
              tunnel: w349 -> [w356 _]
              tunnel: [w355 _] -> w348
              tunnel: [w354 _] -> w335
              frame No Error {
                n204 = call-poly <vilib>:"Read Delimited Spreadsheet.vi"("file path (dialog if empty)"=w356, "format (%.3f)"="%.9f", "transpose? (F)"=TRUE) -> ("new file path (Not A Path if cancelled)"=w355:path, "first row"=w354:dbl[])  [unwired: 7 in, 4 out]
              }
              frame Error {
              }
            }
            n205 = Strip Path(path=w348) -> (name=w347:string)  [unwired: 1 out]
            n206 = Absolute Value(x=w335) -> (abs(x)=w341:dbl[])
            n207 = Match Pattern(string=w347, regular expression=w342) -> (before substring=w346:string, after substring=w344:string)  [unwired: 1 in, 2 out]
            n208 = property on="Waveform Graph" class="WFGraph (strict)"("Value"=w335) -> (error out=w334:errorcluster)  [unwired: 2 in, 1 out]
            n209 = Array Max & Min(array=w341) -> (max value=w340:dbl)  [unwired: 3 out]
            n210 = Match Pattern(string=w344, regular expression=w342) -> (before substring=w343:string)  [unwired: 1 in, 3 out]
            n211 = Fract/Exp String To Number(string=w346) -> (number=w345:dbl)  [unwired: 3 in, 1 out]
            n212 = Multiply(x=1.3, y=w340) -> (x*y=w337:dbl)
            n213 = Negate(x=w337) -> (-x=w338:dbl)
            n214 = Fract/Exp String To Number(string=w343) -> (number=w333:dbl)  [unwired: 3 in, 1 out]
            n215 = property on="Waveform Graph" class="WFGraph (strict)"(error in=w334, "YScale.Maximum"=w337, "YScale.Minimum"=w338) -> ()  [unwired: 1 in, 2 out]
            n216 = local write "信号幅值[V]"(w333) -> ()
            n217 = local write "起始频率[Hz]"(w345) -> ()
          }
        }
        n218 = Insert Into Array(array=w294, new element="apply" ("new element/subarray")) -> (w295:string[])  [unwired: 1 in]
      }
      frame "Exit" {
      }
      frame "Init" {
        w373 = FALSE ("Stop")
        w368 = 44100 ("Rate")
        n219 = call <vilib>:"Application Directory.vi"() -> ("Application Directory"=w386:path)
        n220 = Build Path(base path=w386, name or relative path="main.dat" ("名称或相对路径")) -> (appended path=w385:path)
        n221 = call "File Read Binary File.vi"("file path"=w385) -> ("error Output"=w384:errorcluster, "Variant Output"=w383:variant)  [unwired: 8 in, 1 out]
        n222 = local write "Stop"(w373) -> ()
        n223 = local write "开始测试"(w373) -> ()
        n224 = property on="开始测试" class="Bool (strict)"("Visible"=TRUE, "Value"=FALSE ("开始测试")) -> ()  [unwired: 2 in, 2 out]
        n225 = local write "应用"(FALSE ("应用")) -> ()
        n226 = case shown="No Error" w384 {
          tunnel: w383 -> [w397 _]
          tunnel: [w396 _] -> w382
          frame No Error {
            n227 = Variant To Data(type=T5 {"起始频率"=0.0, "终止频率"=0.0, "信号幅值"=0.0, "信号时长"=0.0, "重复次数"=3, "扫频模式"=TRUE}, Variant=w397) -> (data=w396:T5)  [unwired: 1 in, 1 out]
          }
          frame Error {
          }
        }
        n228 = Reciprocal(x=w368) -> (1/x=w367:dbl)
        n229 = property on="Waveform Graph" class="WFGraph (strict)"("XScale.Multiplier"=w367) -> ()  [unwired: 2 in, 2 out]
        n230 = Bundle By Name(cluster=cluster{"Rate":i32, "Bits":i32, "Channels":u32} {"Rate"=48000, "Bits"=16, "Channels"=2} ("Format"), "Rate"=w368, "Bits"=24, "Channels"=u32 2) -> (→"format":cluster{"Rate":i32, "Bits":i32, "Channels":u32})
        n231 = Unbundle By Name(w382) -> ("起始频率"=w381:dbl, "终止频率"=w380:dbl, "信号幅值"=w379:dbl, "信号时长"=w378:dbl, "扫频模式"=w366:bool)
        n232 = local write "Buffer"(T1 {"# buffers"=4, "Buffer size"=2048, "unit (ms)"=enum."Samples"} ("Buffer")) -> ()
        n233 = local write "单次信号时长[s]"(w378) -> ()
        n234 = local write "信号幅值[V]"(w379) -> ()
        n235 = local write "起始频率[Hz]"(w381) -> ()
        n236 = local write "终止频率[Hz]"(w380) -> ()
        n237 = global write "Global.vi" "扫频模式"(w366) -> ()
        n238 = case shown="True" w366 {
          frame False {
            n239 = property on="单次信号时长[s]" class="DigNum (strict)"("Visible"=FALSE) -> ()  [unwired: 2 in, 2 out]
            n240 = property on="终止频率[Hz]" class="DigNum (strict)"("Visible"=FALSE) -> ()  [unwired: 2 in, 2 out]
            n241 = property on="起始频率[Hz]" class="DigNum (strict)"("Caption.Text"="单频频率[Hz]") -> ()  [unwired: 2 in, 2 out]
          }
          frame True {
            n242 = property on="单次信号时长[s]" class="DigNum (strict)"("Visible"=TRUE) -> ()  [unwired: 2 in, 2 out]
            n243 = property on="终止频率[Hz]" class="DigNum (strict)"("Visible"=TRUE) -> ()  [unwired: 2 in, 2 out]
            n244 = property on="起始频率[Hz]" class="DigNum (strict)"("Caption.Text"="起始频率[Hz]") -> ()  [unwired: 2 in, 2 out]
          }
        }
        n245 = property on="Waveform Graph" class="WFGraph (strict)"("Visible"=TRUE) -> ()  [unwired: 2 in, 2 out]
        n246 = Two Button Dialog(message="请选择机型", 1:"其它" ("F button name (\"Cancel\")"), 2:"有源音箱" ("T button name (\"OK\")")) -> (T button?=w361:bool)
        n247 = global write "Global.vi" "有源音箱"(w361) -> ()
      }
    }
  }
